vi "Пр01.vi"() -> ()   [LabVIEW 2011]
panel:
  in  "Нижній max":dbl
  in  "Верхній max":dbl
  in  "Верхній min":dbl
  in  "Нижній min":dbl
  out "Результати (0 та 1)":u8(graph)
  out "Отримане число":dbl
  in  "stop":bool
  in  "Генерувати":bool
  # "Обати діапазони чисел:"
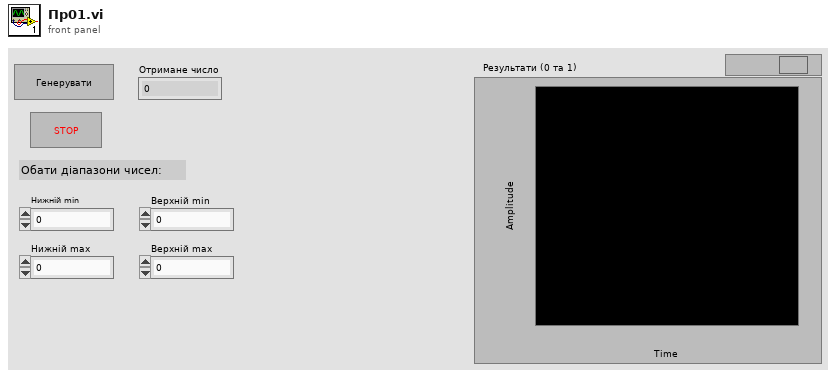
[diagram p1: front panel]
types:
  T1 = typedef "ПР01 Контрол.ctl" = enum16{"min1", "min2", "max1", "max2"}
  T2 = cluster{"min1":dbl, "min2":dbl, "max1":dbl, "max2":dbl, "Найбільше":dbl}
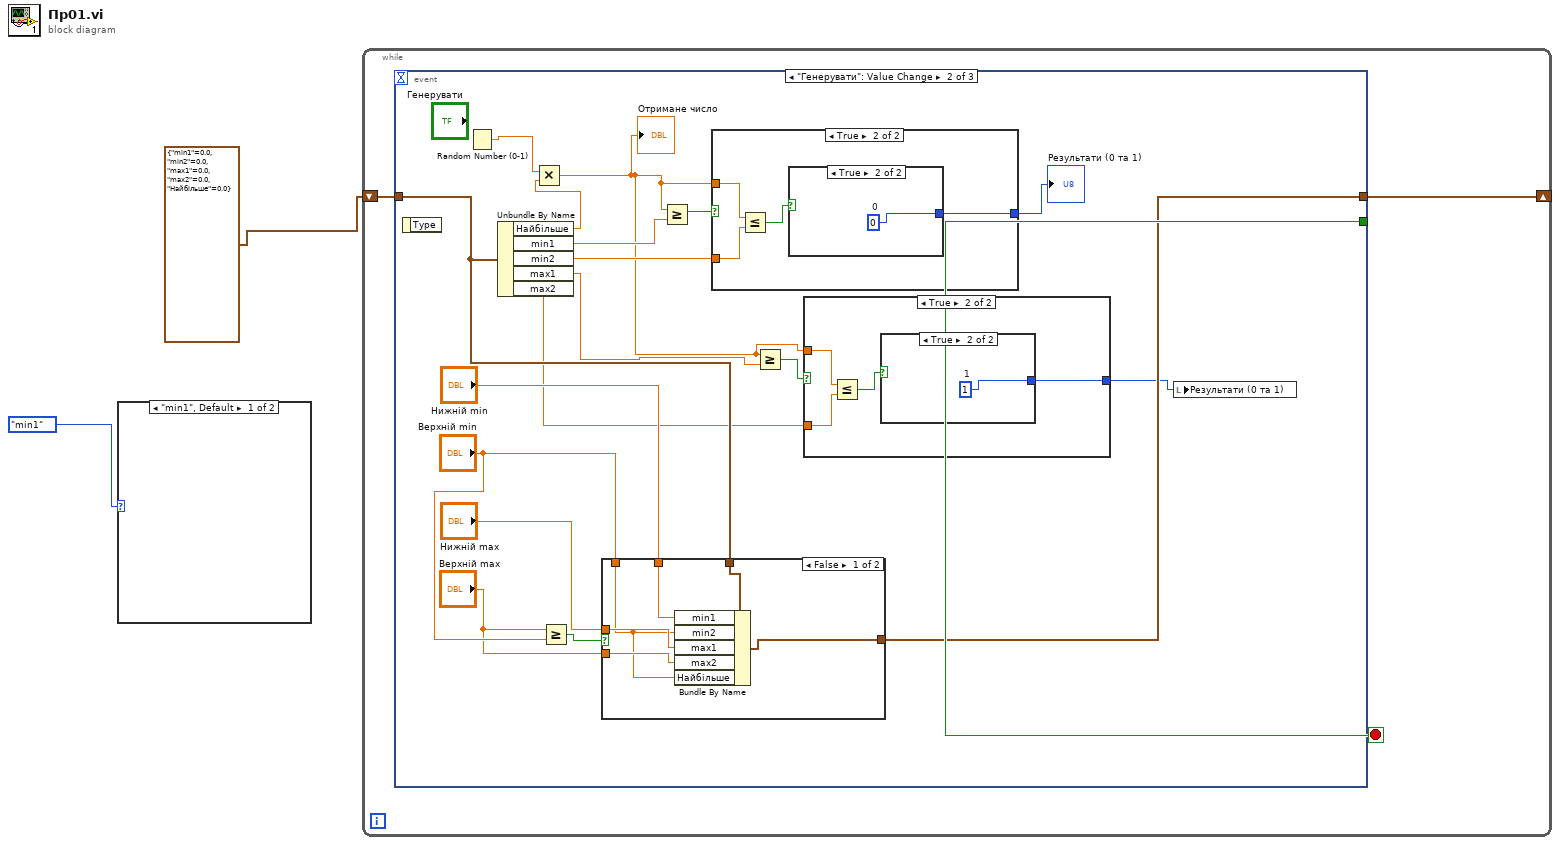
[diagram p0: block diagram]
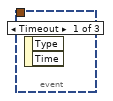
[diagram p3: hidden frame]
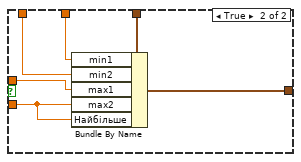
[diagram p6: hidden frame]
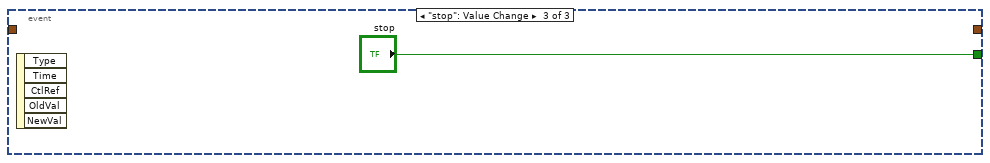
[diagram p9: hidden frame]
diagram:
  n1 = case shown="\"min1\", Default" ПР01_Контрол."min1" ("Enum") {
    frame "min1", Default {
    }
    frame "min2" {
    }
  }
  n2 = while {
    shift-right: [w3] -> _
    shift-left: T2 {"min1"=0.0, "min2"=0.0, "max1"=0.0, "max2"=0.0, "Найбільше"=0.0} -> [w4]
    stop <- w5 stop-if-true
    n3 = event shown="[1] \"Генерувати\": Value Change" {
      selector: _ -> [_ _ _]
      dyn-events: _ -> [_ _ _]
      timeout: _ -> [_ _ _]
      tunnel: [_ _ "stop"] -> w5
      tunnel: w4 -> [_ w16 _]
      tunnel: [_ w22 _] -> w3
      event Timeout {
        n4 = event-data() -> ()  [unwired: 1 in, 2 out]
      }
      event "Генерувати": Value Change {
        n5 = event-data() -> ()  [unwired: 1 in, 1 out]
        n6 = Random Number (0-1)() -> (number: 0 to 1=w17:dbl)
        n7 = Unbundle By Name(w16) -> ("Найбільше"=w15:dbl, "min1"=w14:dbl, "min2"=w12:dbl, "max1"=w9:dbl, "max2"=w7:dbl)
        n8 = Multiply(x=w17, y=w15) -> (x*y=w8:dbl)
        "Отримане число" <- w8
        n9 = Greater Or Equal?(x="Верхній max", y="Верхній min") -> (x >= y?=w23:bool)
        n10 = case shown="False" w23 {
          tunnel: w16 -> [w30 w40]
          tunnel: [w29 w39] -> w22
          tunnel: "Нижній min" -> [w34 w38]
          tunnel: "Верхній min" -> [w31 w37]
          tunnel: "Нижній max" -> [w33 w36]
          tunnel: "Верхній max" -> [w32 w35]
          frame False {
            n11 = Bundle By Name(cluster=w30, "min1"=w34, "min2"=w31, "max1"=w33, "max2"=w32, "Найбільше"=w31) -> (w29:T2)
          }
          frame True {
            n12 = Bundle By Name(cluster=w40, "min1"=w38, "min2"=w37, "max1"=w36, "max2"=w35, "Найбільше"=w35) -> (w39:T2)
          }
        }
        n13 = Greater Or Equal?(x=w8, y=w14) -> (x >= y?=w13:bool)
        n14 = case shown="True" w13 {
          tunnel: w8 -> [_ w44]
          tunnel: w12 -> [_ w43]
          tunnel: [_ w41] -> w11
          frame False {
          }
          frame True {
            n15 = Less Or Equal?(x=w44, y=w43) -> (x <= y?=w42:bool)
            n16 = case shown="True" w42 {
              tunnel: [_ w45] -> w41
              frame False {
              }
              frame True {
                w45 = u8 0  # 0
              }
            }
          }
        }
        "Результати (0 та 1)" <- w11
        n17 = Greater Or Equal?(x=w8, y=w9) -> (x >= y?=w10:bool)
        n18 = case shown="True" w10 {
          tunnel: w8 -> [_ w27]
          tunnel: w7 -> [_ w26]
          tunnel: [_ w24] -> w6
          frame False {
          }
          frame True {
            n19 = Less Or Equal?(x=w27, y=w26) -> (x <= y?=w25:bool)
            n20 = case shown="True" w25 {
              tunnel: [_ w28] -> w24
              frame False {
              }
              frame True {
                w28 = u8 1  # 1
              }
            }
          }
        }
        n21 = local write "Результати (0 та 1)"(w6) -> ()
      }
      event "stop": Value Change {
        n22 = event-data() -> ()  [unwired: 1 in, 5 out]
      }
    }
  }
